vi "Log_MessageHandler_LoadLastLogFile.vi"(8 "error in":errorcluster, 11 "MessageHandler in":refnum<class "MessageHandler.lvclass">) -> (0 "error out":errorcluster, 3 "MessageHandler out":refnum<class "MessageHandler.lvclass">)   [LabVIEW 2013, in "MessageHandler.lvclass"]
uses:
  MessageHandler.lvclass
  MessageHandler.lvclass/MessageHandler.ctl
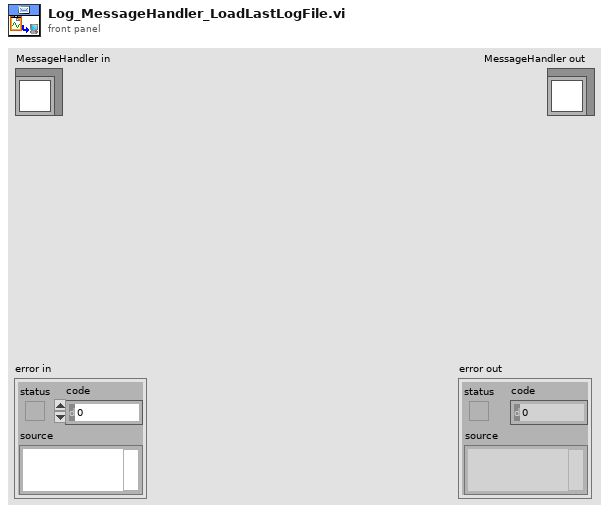
[diagram p1: front panel]
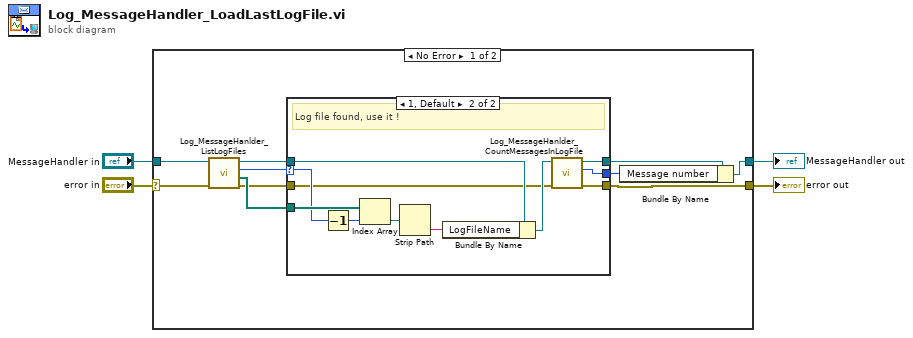
[diagram p0: block diagram]
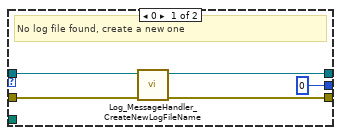
[diagram p2: hidden frame]
diagram:
  n1 = case shown="No Error" "error in" {
    selector: "error in" -> [w14 w32]
    tunnel: [w6 w32] -> w3
    tunnel: [w7 w31] -> w1
    tunnel: "MessageHandler in" -> [w11 w31]
    frame No Error {
      n2 = call-dynamic "Log_MessageHanlder_ListLogFiles.vi"("error in (no error)"=w14, "MessageHandler in"=w11) -> ("error out"=w9:errorcluster, "Log file paths"=w12:path[], "Log file nb"=w13:u32, "MessageHandler out"=w10:refnum<class "MessageHandler.lvclass">)  [unwired: 6 in]
      n3 = case shown="1, Default" w13 {
        selector: w13 -> [_ w29]
        tunnel: w12 -> [_ w30]
        tunnel: [w17 w25] -> w8
        tunnel: w10 -> [w18 w24]
        tunnel: [w16 w26] -> w6
        tunnel: w9 -> [w19 w21]
        tunnel: [u32 0 ("Message number") w20] -> w5
        frame 0 {
          # "No log file found, create a new one"
          n4 = call-dynamic "Log_MessageHandler_CreateNewLogFileName.vi"("error in (no error)"=w19, "MessageHandler in"=w18) -> ("error out"=w16:errorcluster, "MessageHandler out"=w17:refnum<class "MessageHandler.lvclass">)  [unwired: 8 in]
        }
        frame 1, Default {
          # "Log file found, use it !"
          n5 = Decrement(x=w29) -> (x-1=w28:u32)
          n6 = Index Array(array=w30, index=w28) -> (element=w27:path)
          n7 = Strip Path(path=w27) -> (name=w23:string)  [unwired: 1 out]
          n8 = Bundle By Name(cluster=w24, "LogFileName"=w23) -> (w22:refnum<class "MessageHandler.lvclass">)
          n9 = call-dynamic "Log_MessageHanlder_CountMessagesInLogFile.vi"("error in"=w21, "MessageHandler in"=w22) -> ("error out"=w26:errorcluster, "NbMessages"=w20:i32, "MessageHandler out"=w25:refnum<class "MessageHandler.lvclass">)  [unwired: 7 in]
        }
      }
      n10 = Bundle By Name(cluster=w8, "Message number"=w5) -> (w7:refnum<class "MessageHandler.lvclass">)
    }
    frame Error {
    }
  }
  "error out" <- w3
  "MessageHandler out" <- w1
